vi "what.vi"() -> ()   [LabVIEW 2017]
uses:
  what.ctl
panel:
  out "Counter Value":dbl
  out "index of element":i32
  in  "Abort":bool
  in  "Run Through":bool
  in  "Floor 3":bool
  in  "Floor 2":bool
  in  "Floor 1":bool
  in  "stop":bool
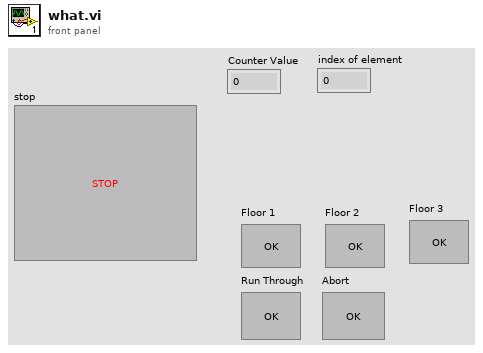
[diagram p1: front panel]
types:
  T1 = typedef "what.ctl" = enum16{"Initialize", "Floor 1", "Floor 2", "Floor 3", "GO!", "Stop!", "Wait for User Input"}
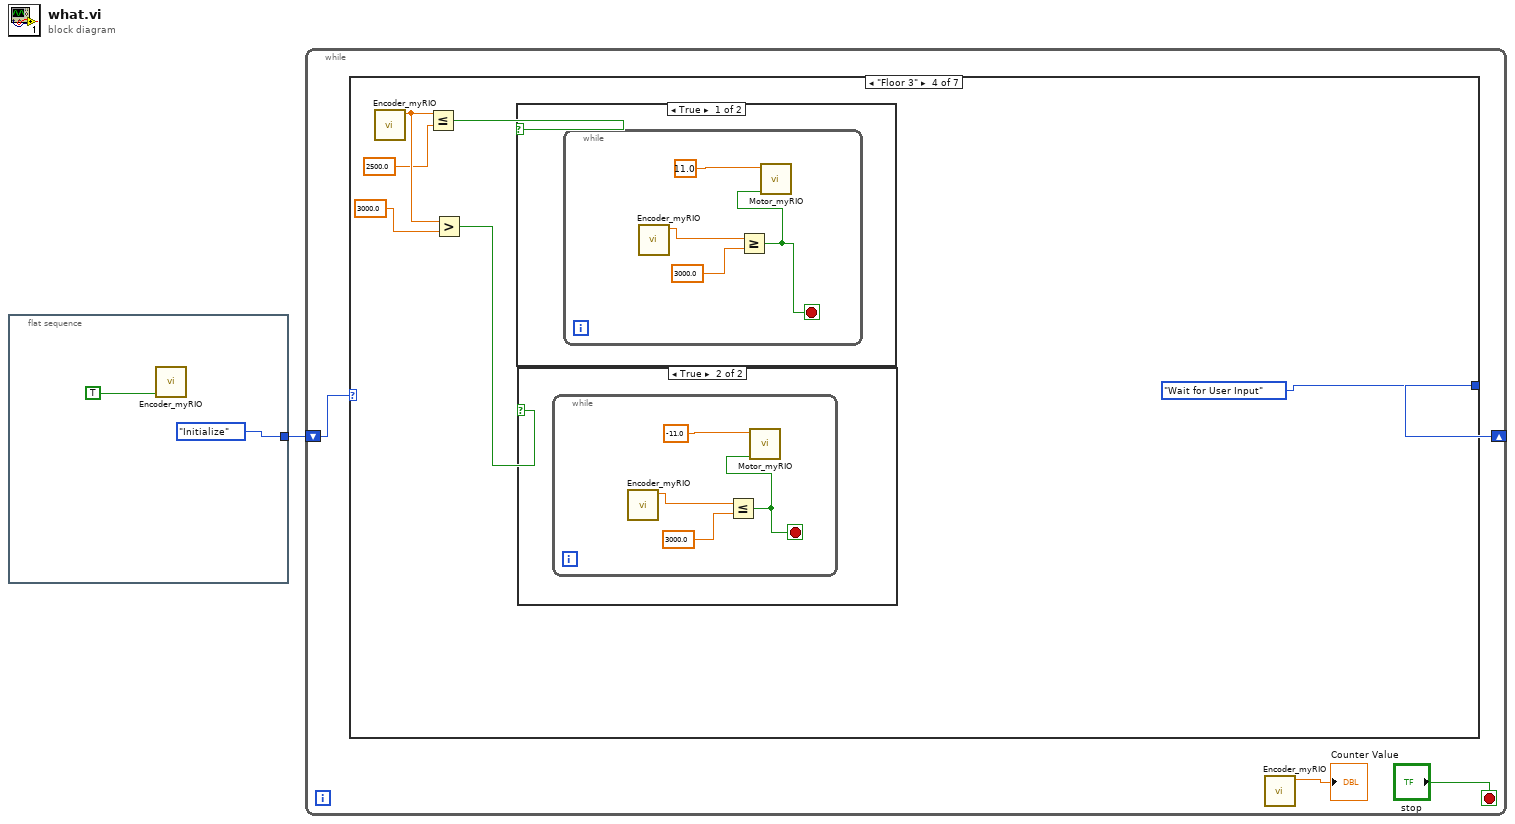
[diagram p0: block diagram]
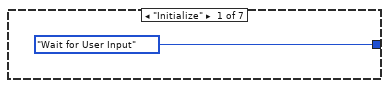
[diagram p2: hidden frame]
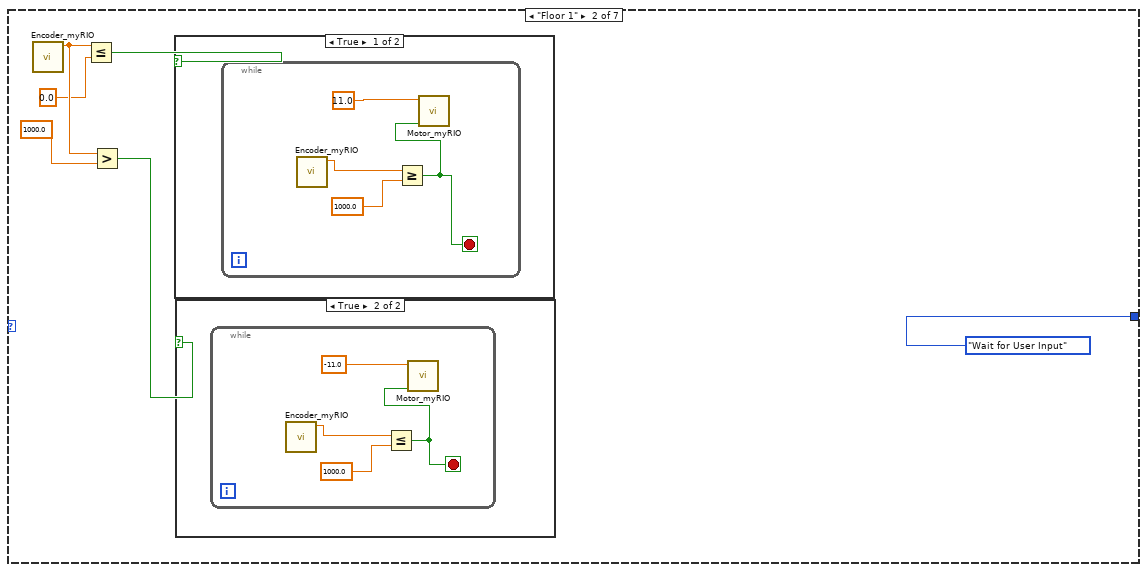
[diagram p3: hidden frame]
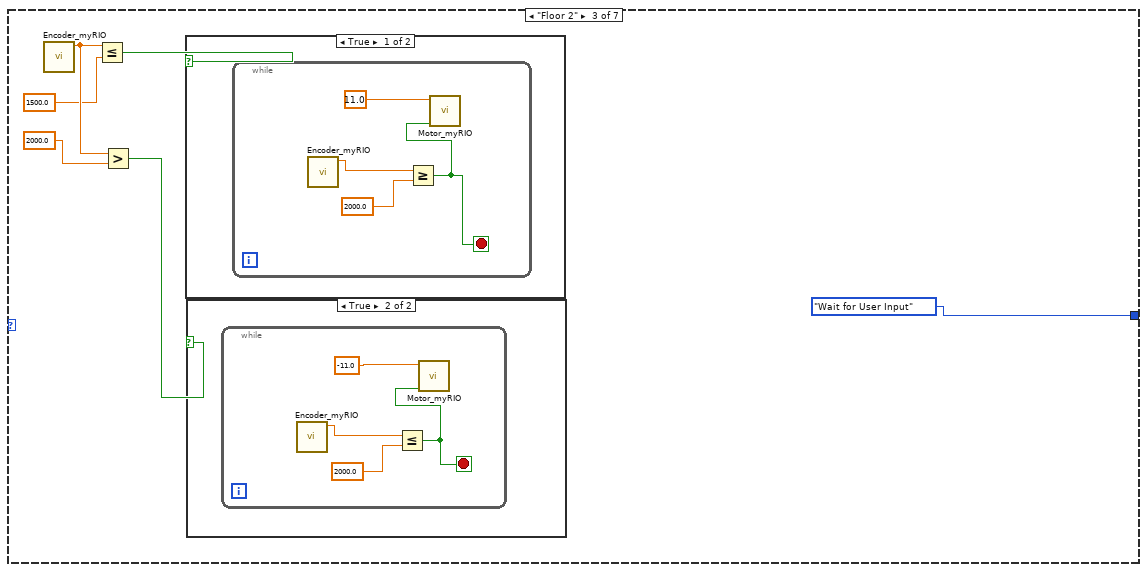
[diagram p6: hidden frame]
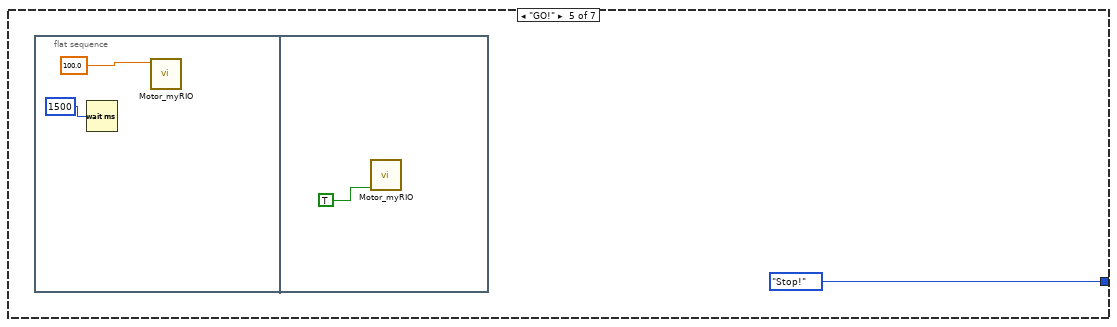
[diagram p11: hidden frame]
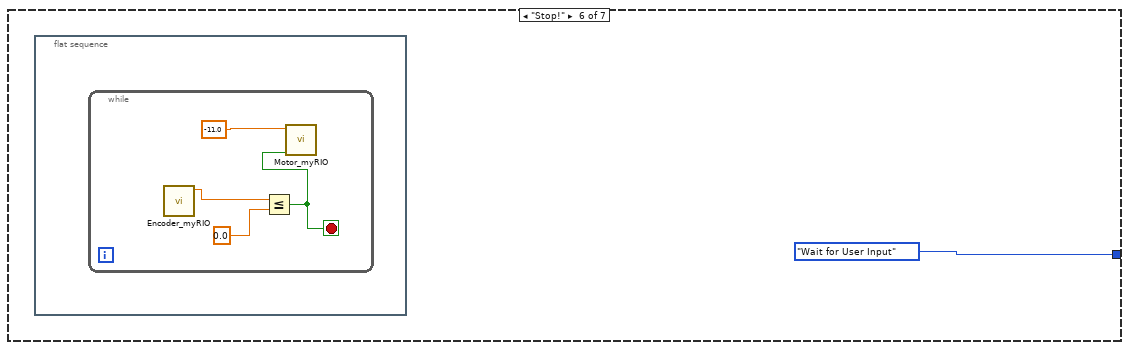
[diagram p12: hidden frame]
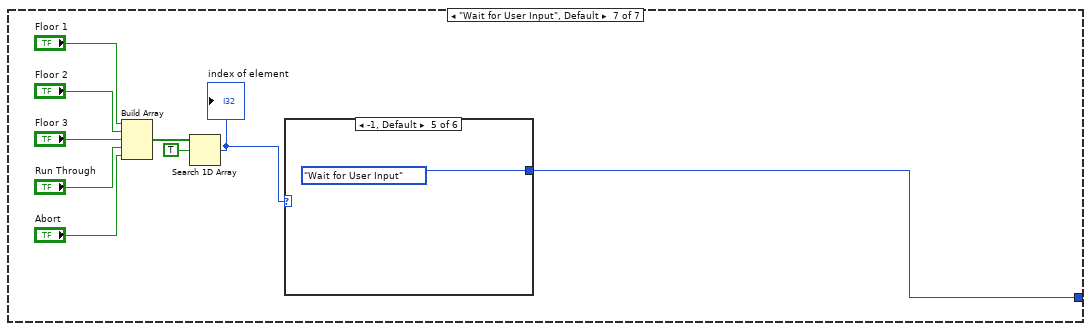
[diagram p13: hidden frame]
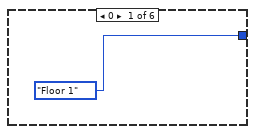
[diagram p14: hidden frame]
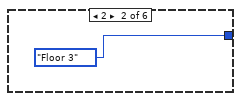
[diagram p15: hidden frame]
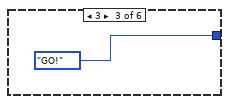
[diagram p16: hidden frame]
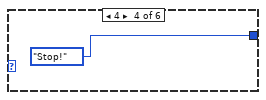
[diagram p17: hidden frame]
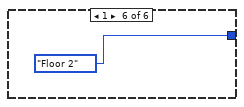
[diagram p18: hidden frame]
diagram:
  n1 = flat-sequence {
    tunnel: [what."Initialize"] -> w1
    frame #0 {
      n2 = call "Encoder_myRIO.vi"("Reset"=TRUE) -> ()  [unwired: 9 in, 2 out]
    }
  }
  n3 = while {
    shift-right: [w7] -> _
    shift-left: w1 -> [w4]
    stop <- "stop" stop-if-true
    n4 = case shown="\"Floor 3\"" w4 {
      tunnel: [what."Wait for User Input" what."Wait for User Input" what."Wait for User Input" what."Wait for User Input" what."Stop!" what."Wait for User Input" w60] -> w7
      frame "Initialize" {
      }
      frame "Floor 1" {
        n5 = call "Encoder_myRIO.vi"() -> ("Counter Value"=w11:dbl)  [unwired: 10 in, 1 out]
        n6 = Less Or Equal?(x=w11, y=0.0) -> (x <= y?=w13:bool)
        n7 = Greater?(x=w11, y=1000.0) -> (0:w12:bool)
        n8 = case shown="True" w13 {
          frame True {
            n9 = while {
              stop <- w15 stop-if-true
              n10 = call "Encoder_myRIO.vi"() -> ("Counter Value"=w18:dbl)  [unwired: 10 in, 1 out]
              n11 = Greater Or Equal?(x=w18, y=1000.0) -> (x >= y?=w15:bool)
              n12 = call "Motor_myRIO.vi"("Stop VI"=w15, "Duty Cycle (-100 to +100)"=11.0) -> ()  [unwired: 10 in]
            }
          }
          frame False {
          }
        }
        n13 = case shown="True" w12 {
          frame False {
          }
          frame True {
            n14 = while {
              stop <- w19 stop-if-true
              n15 = call "Encoder_myRIO.vi"() -> ("Counter Value"=w22:dbl)  [unwired: 10 in, 1 out]
              n16 = Less Or Equal?(x=w22, y=1000.0) -> (x <= y?=w19:bool)
              n17 = call "Motor_myRIO.vi"("Stop VI"=w19, "Duty Cycle (-100 to +100)"=-11.0) -> ()  [unwired: 10 in]
            }
          }
        }
      }
      frame "Floor 2" {
        n18 = call "Encoder_myRIO.vi"() -> ("Counter Value"=w25:dbl)  [unwired: 10 in, 1 out]
        n19 = Less Or Equal?(x=w25, y=1500.0) -> (x <= y?=w27:bool)
        n20 = Greater?(x=w25, y=2000.0) -> (0:w26:bool)
        n21 = case shown="True" w27 {
          frame True {
            n22 = while {
              stop <- w29 stop-if-true
              n23 = call "Encoder_myRIO.vi"() -> ("Counter Value"=w32:dbl)  [unwired: 10 in, 1 out]
              n24 = Greater Or Equal?(x=w32, y=2000.0) -> (x >= y?=w29:bool)
              n25 = call "Motor_myRIO.vi"("Stop VI"=w29, "Duty Cycle (-100 to +100)"=11.0) -> ()  [unwired: 10 in]
            }
          }
          frame False {
          }
        }
        n26 = case shown="True" w26 {
          frame False {
          }
          frame True {
            n27 = while {
              stop <- w33 stop-if-true
              n28 = call "Encoder_myRIO.vi"() -> ("Counter Value"=w36:dbl)  [unwired: 10 in, 1 out]
              n29 = Less Or Equal?(x=w36, y=2000.0) -> (x <= y?=w33:bool)
              n30 = call "Motor_myRIO.vi"("Stop VI"=w33, "Duty Cycle (-100 to +100)"=-11.0) -> ()  [unwired: 10 in]
            }
          }
        }
      }
      frame "Floor 3" {
        n31 = call "Encoder_myRIO.vi"() -> ("Counter Value"=w39:dbl)  [unwired: 10 in, 1 out]
        n32 = Less Or Equal?(x=w39, y=2500.0) -> (x <= y?=w41:bool)
        n33 = Greater?(x=w39, y=3000.0) -> (0:w40:bool)
        n34 = case shown="True" w41 {
          frame True {
            n35 = while {
              stop <- w43 stop-if-true
              n36 = call "Encoder_myRIO.vi"() -> ("Counter Value"=w46:dbl)  [unwired: 10 in, 1 out]
              n37 = Greater Or Equal?(x=w46, y=3000.0) -> (x >= y?=w43:bool)
              n38 = call "Motor_myRIO.vi"("Stop VI"=w43, "Duty Cycle (-100 to +100)"=11.0) -> ()  [unwired: 10 in]
            }
          }
          frame False {
          }
        }
        n39 = case shown="True" w40 {
          frame False {
          }
          frame True {
            n40 = while {
              stop <- w47 stop-if-true
              n41 = call "Encoder_myRIO.vi"() -> ("Counter Value"=w50:dbl)  [unwired: 10 in, 1 out]
              n42 = Less Or Equal?(x=w50, y=3000.0) -> (x <= y?=w47:bool)
              n43 = call "Motor_myRIO.vi"("Stop VI"=w47, "Duty Cycle (-100 to +100)"=-11.0) -> ()  [unwired: 10 in]
            }
          }
        }
      }
      frame "GO!" {
        n44 = flat-sequence {
          frame #0 {
            n45 = Wait (ms)(milliseconds to wait=u32 1500) -> ()  [unwired: 1 out]
            n46 = call "Motor_myRIO.vi"("Duty Cycle (-100 to +100)"=100.0) -> ()  [unwired: 11 in]
          }
          frame #1 {
            n47 = call "Motor_myRIO.vi"("Stop VI"=TRUE) -> ()  [unwired: 11 in]
          }
        }
      }
      frame "Stop!" {
        n48 = flat-sequence {
          frame #0 {
            n49 = while {
              stop <- w56 stop-if-true
              n50 = call "Encoder_myRIO.vi"() -> ("Counter Value"=w59:dbl)  [unwired: 10 in, 1 out]
              n51 = Less Or Equal?(x=w59, y=0.0) -> (x <= y?=w56:bool)
              n52 = call "Motor_myRIO.vi"("Stop VI"=w56, "Duty Cycle (-100 to +100)"=-11.0) -> ()  [unwired: 10 in]
            }
          }
        }
      }
      frame "Wait for User Input", Default {
        n53 = Build Array("Floor 1", "Floor 2", "Floor 3", "Run Through", "Abort") -> (w68:bool[])
        n54 = Search 1D Array(1D array=w68, element=TRUE) -> (index of element=w61:i32)  [unwired: 1 in]
        "index of element" <- w61
        n55 = case shown="-1, Default" w61 {
          tunnel: [what."Floor 1" what."Floor 3" what."GO!" what."Stop!" what."Wait for User Input" what."Floor 2"] -> w60
          frame 0 {
          }
          frame 2 {
          }
          frame 3 {
          }
          frame 4 {
          }
          frame -1, Default {
          }
          frame 1 {
          }
        }
      }
    }
    n56 = call "Encoder_myRIO.vi"() -> ("Counter Value"=→"Counter Value":dbl)  [unwired: 10 in, 1 out]
  }
